vi "Write Pattern Script.vi"(8 "error in (no error)":errorcluster, 10 "Pattern Script":string, 11 "BML_Frame_Root in":refnum<class "BML_Frame_Root.lvclass">) -> (0 "error out":errorcluster, 3 "BML_Frame_Root out":refnum<class "BML_Frame_Root.lvclass">)   [LabVIEW 2018, in "BML_Frame_Root.lvclass"]
uses:
  BML_Frame_Root.lvclass
  BML_Frame_Root.lvclass/BML_Frame_Root.ctl
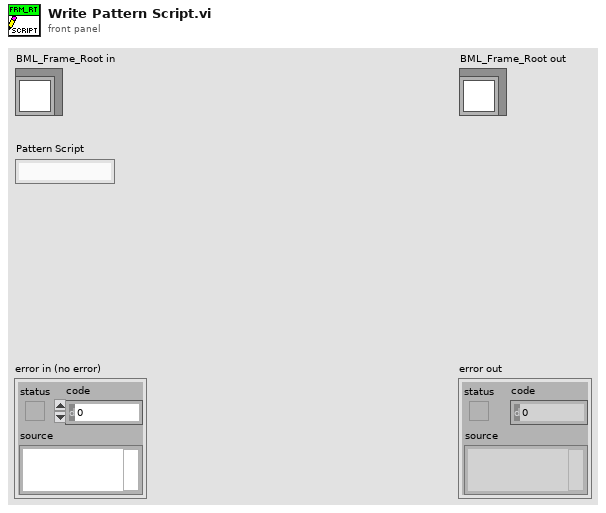
[diagram p1: front panel]
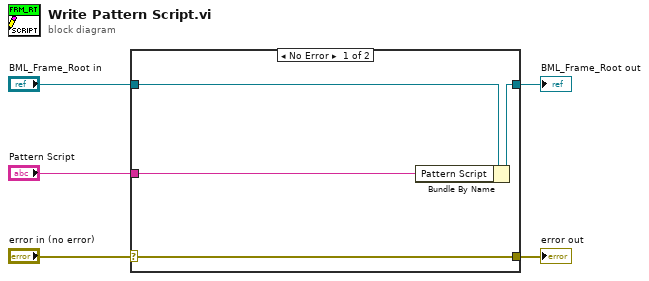
[diagram p0: block diagram]
diagram:
  n1 = case shown="No Error" "error in (no error)" {
    selector: "error in (no error)" -> [w9 w10]
    tunnel: [w9 w10] -> w4
    tunnel: [w7 w11] -> w2
    tunnel: "BML_Frame_Root in" -> [w8 w11]
    tunnel: "Pattern Script" -> [w6 _]
    frame No Error {
      n2 = Bundle By Name(cluster=w8, "Pattern Script"=w6) -> (w7:refnum<class "BML_Frame_Root.lvclass">)
    }
    frame Error {
    }
  }
  "error out" <- w4
  "BML_Frame_Root out" <- w2
